vi "Determine Closest Point Indices.vi"(10 "Range":i32[](array[numeric]), 11 "Coordinates":i32[][](array[numeric])) -> (3 "Closest Point Indices":i32[][](array[numeric]))   [LabVIEW 2019]
doc: "At each given point, find the minimum manhattan distance and output that index."
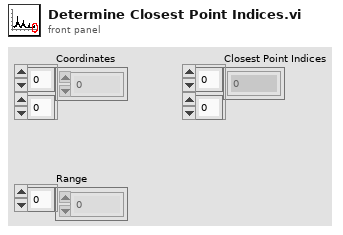
[diagram p1: front panel]
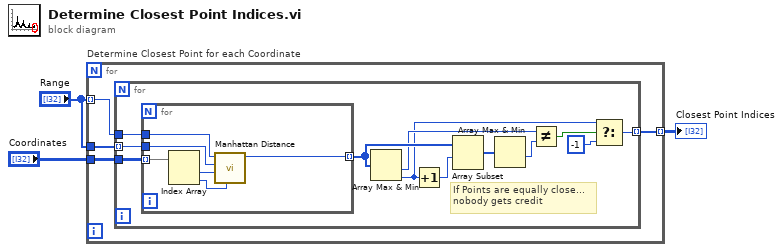
[diagram p0: block diagram]
diagram:
  n1 = for "Determine Closest Point for each Coordinate" {
    tunnel: "Range" -> [w6] mode=indexing
    tunnel: "Range" -> [w7]
    tunnel: "Coordinates" -> [w5]
    tunnel: [w4] -> w1 mode=indexing
    n2 = for {
      tunnel: w7 -> [w18] mode=indexing
      tunnel: w6 -> [w17]
      tunnel: w5 -> [w19]
      tunnel: [w10] -> w4 mode=indexing
      # "If Points are equally close...\nnobody gets credit"
      n3 = for {
        tunnel: w19 -> [w25] mode=indexing
        tunnel: w18 -> [w21]
        tunnel: w17 -> [w22]
        tunnel: [w20] -> w16 mode=indexing
        n4 = Index Array(array=w25) -> (element #1=w24:i32, element #2=w23:i32)  [unwired: 2 in]
        n5 = call "Manhattan Distance.vi"("y 2"=w23, "x 2"=w24, "x"=w21, "y"=w22) -> ("Manhattan Distance"=w20:i32)  [unwired: 7 in]
      }
      n6 = Array Max & Min(array=w16) -> (min value=w14:i32, min index (indices)=w9:i32)  [unwired: 2 out]
      n7 = Increment(x=w9) -> (x+1=w8:i32)
      n8 = Array Subset(array=w16, index=w8) -> (w15:i32[])  [unwired: 1 in]
      n9 = Array Max & Min(array=w15) -> (min value=w13:i32)  [unwired: 3 out]
      n10 = Not Equal?(x=w14, y=w13) -> (x != y?=w12:bool)
      n11 = Select(t=w9, s=w12, f=-1) -> (s? t:f=w10:i32)
    }
  }
  "Closest Point Indices" <- w1
